vi "Initialize.vi"(8 "error in (no error)":errorcluster, 11 "Simulated Interlocks in":refnum<class "Simulated Interlocks.lvclass">) -> (0 "error out":errorcluster, 3 "Simulated Interlocks out":refnum<class "Simulated Interlocks.lvclass">)   [LabVIEW 2020, in "Simulated Interlocks.lvclass"]
uses:
  Simulated Interlocks.lvclass
  Door Interlocks/Interlock Values.ctl
  Door Interlocks/Mode of Operation.ctl
  Simulated Interlocks.lvclass/Simulated Interlocks.ctl
  Door Controller/Door Controller/Simulated Values.vi
  Door Interlocks/Door Interlocks.lvclass
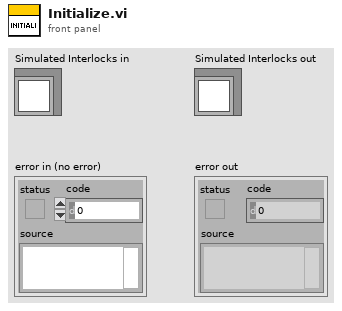
[diagram p1: front panel]
types:
  T1 = typedef "Door Interlocks.lvclass/Interlock Values.ctl" = cluster{"Door Open":bool, "Door Closed":bool, "Mode of Operation":T2}
  T2 = typedef "Door Interlocks.lvclass/Mode of Operation.ctl" = enum16{"Standard", "Interlock Override"}
  T3 = enum32{"Invalid", "Standard", "Closed", "Hidden", "Minimized", "Maximized"}
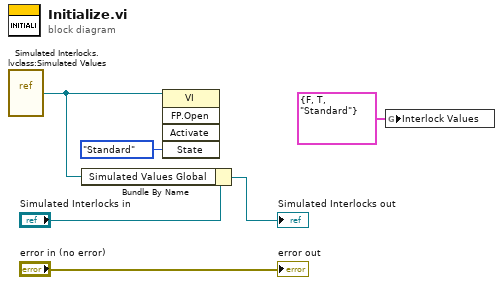
[diagram p0: block diagram]
diagram:
  n1 = vi-ref "Simulated Interlocks.lvclass:Simulated Values.vi"() -> (w3:refnum<vi>)
  n2 = Bundle By Name(cluster="Simulated Interlocks in", "Simulated Values Global"=w3) -> (→"Simulated Interlocks out":refnum<class "Simulated Interlocks.lvclass">)
  n3 = invoke class="VI" method="FP.Open"(reference=w3, "State"=T3."Standard") -> ()  [unwired: 3 in, 5 out]
  n4 = global write "Simulated Values.vi" "Interlock Values"(T1 {"Door Open"=FALSE, "Door Closed"=TRUE, "Mode of Operation"=enum."Standard"} ("Interlock Values")) -> ()
  "error out" <- "error in (no error)"
